vi "SEH Error Notification.vi"(6 "Configuration":T2, 7 "Command":T3, 8 "Error to Send":errorcluster, 11 "Priority":i32) -> (0 "Transmission Error":errorcluster, 1 "Transmitted Error":errorcluster, 2 "Empty?":bool, 3 "Priority Out":i32, 4 "Occurrences":i32, 5 "First Occurrence":timestamp)   [LabVIEW 2014]
uses:
  Controls/Shared/SEH Error Notification Command.ctl
  Controls/Shared/SEH Error Notification Config.ctl
  Controls/SEH/SEH Error Notification Data.ctl
  Controls/Shared/SEH Transmit Error Function.ctl
panel:
  out "Read Ptrs":i32[](array[numeric])
  out "Array":T1[][](array[typedef])
  out "Codes":i32[][](array[numeric])
  out "Sizes":i32[](array[numeric])
  out "Write Ptrs":i32[](array[numeric])
  # "Debug"
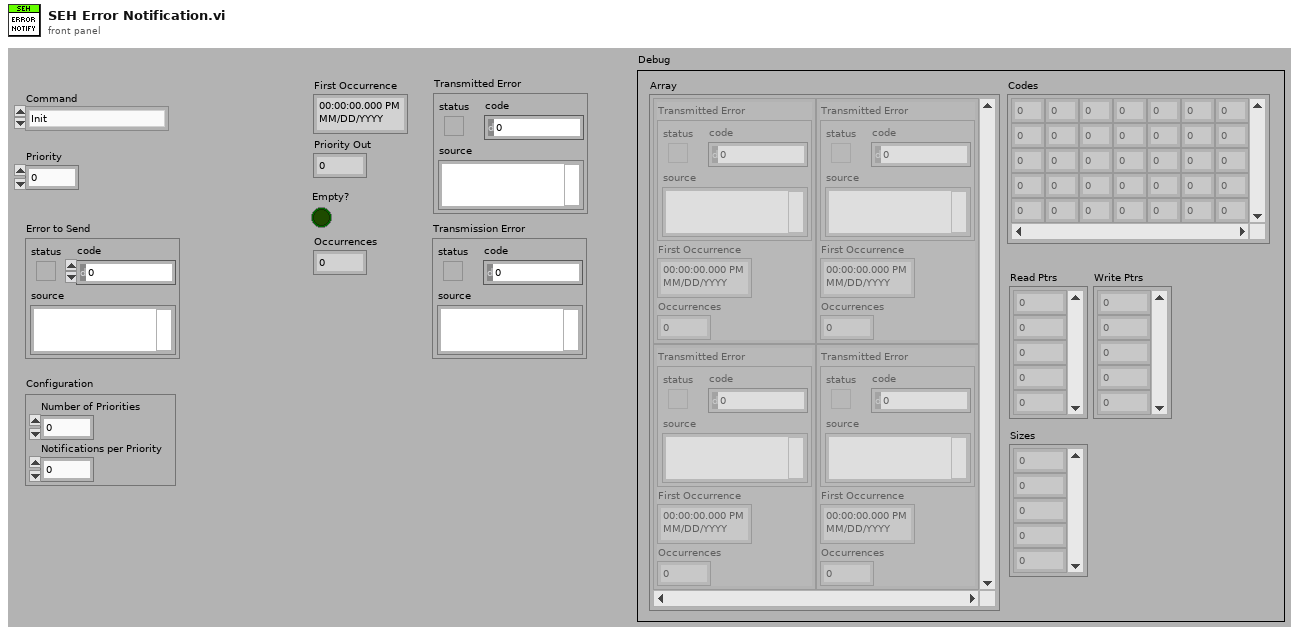
[diagram p1: front panel]
types:
  T1 = typedef "SEH Error Notification Data.ctl" = cluster{"Transmitted Error":errorcluster, "First Occurrence":timestamp, "Occurrences":i32}
  T2 = typedef "SEH Error Notification Config.ctl" = cluster{"Number of Priorities":i32, "Notifications per Priority":i32}
  T3 = typedef "SEH Error Notification Command.ctl" = enum16{"Init", "Send Error", "Check Error", "Invalid Command"}
  T4 = typedef "SEH Transmit Error Function.ctl" = enum8{"Set", "Reset", "No Change"}
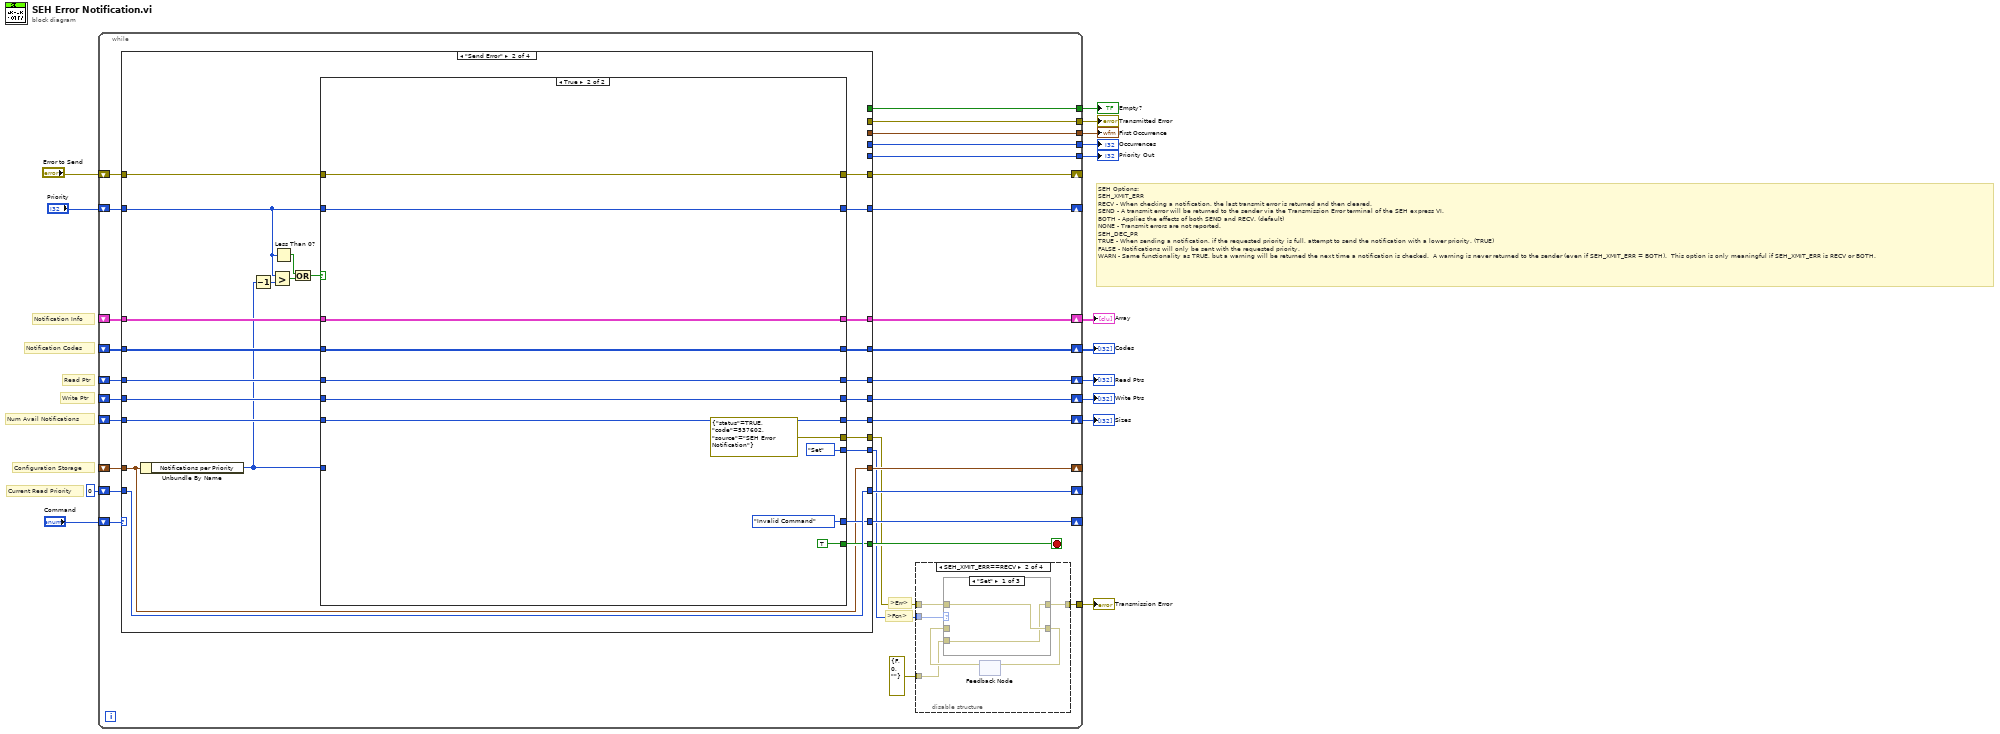
[diagram p0: block diagram]
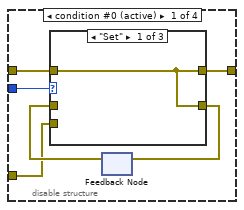
[diagram p2: hidden frame]
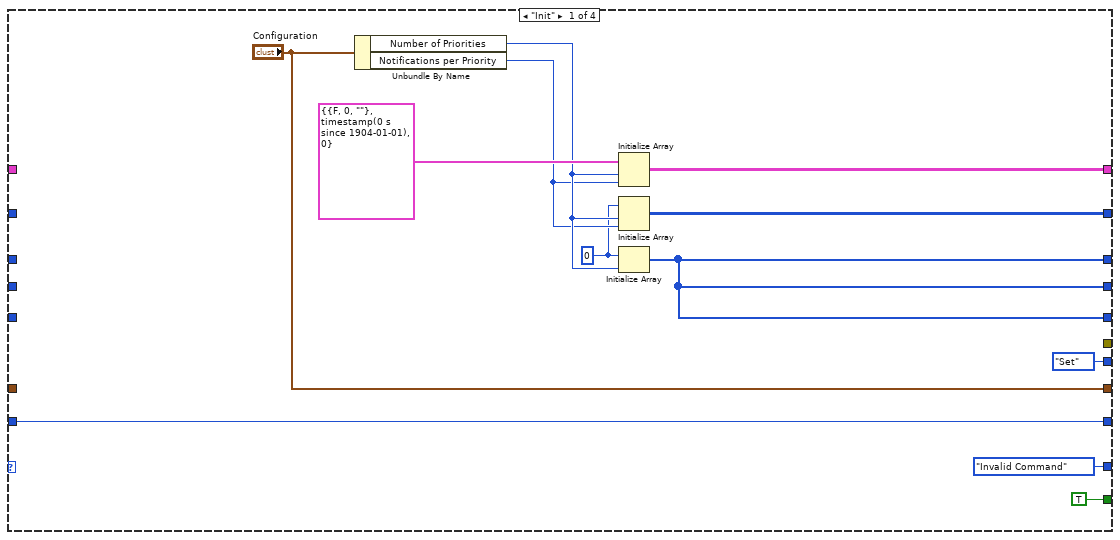
[diagram p9: hidden frame]
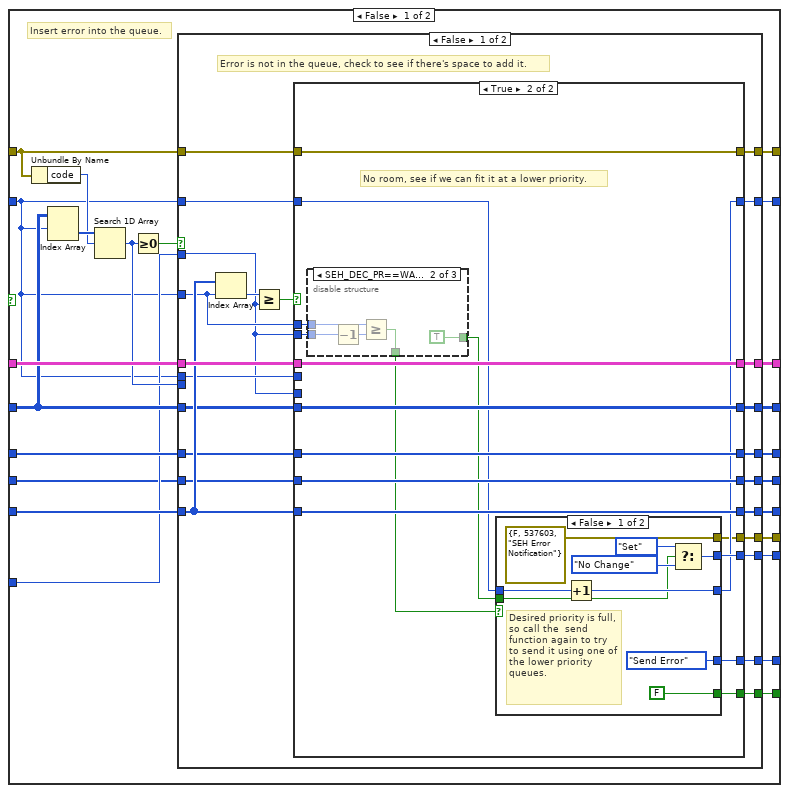
[diagram p10: hidden frame]
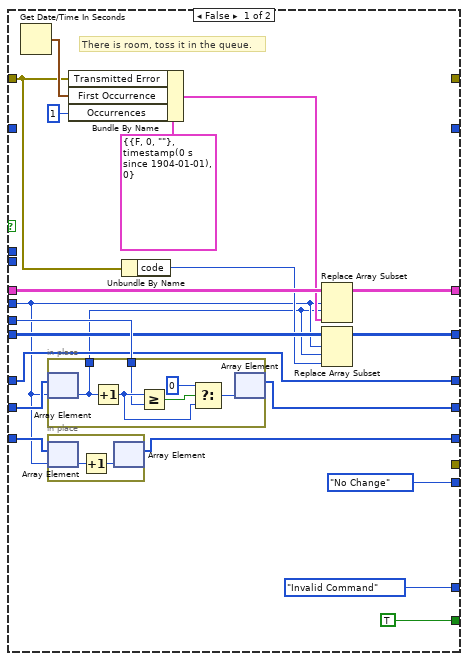
[diagram p11: hidden frame]
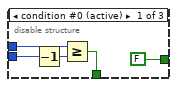
[diagram p12: hidden frame]
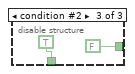
[diagram p13: hidden frame]
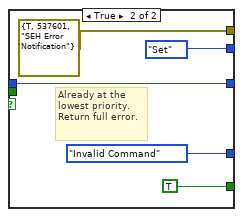
[diagram p14: hidden frame]
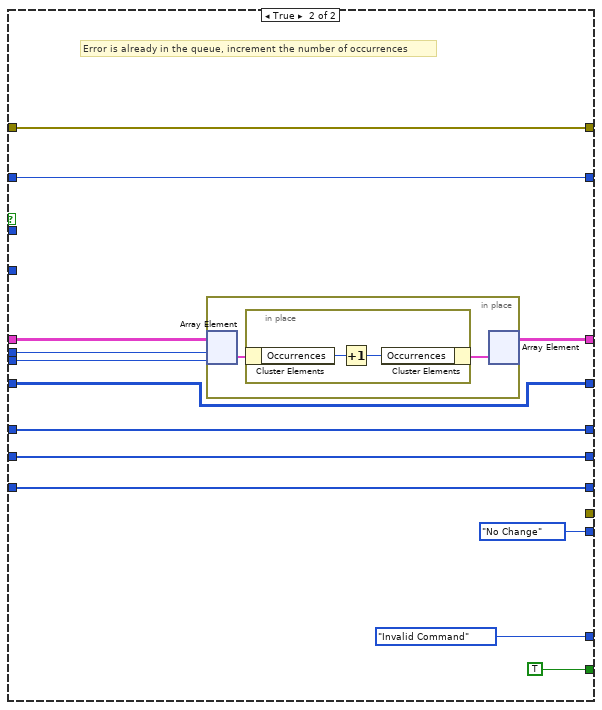
[diagram p15: hidden frame]
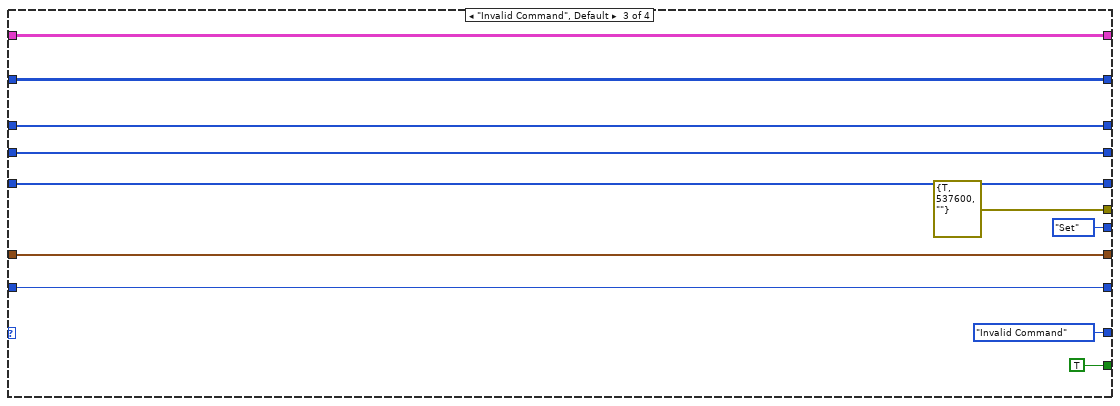
[diagram p16: hidden frame]
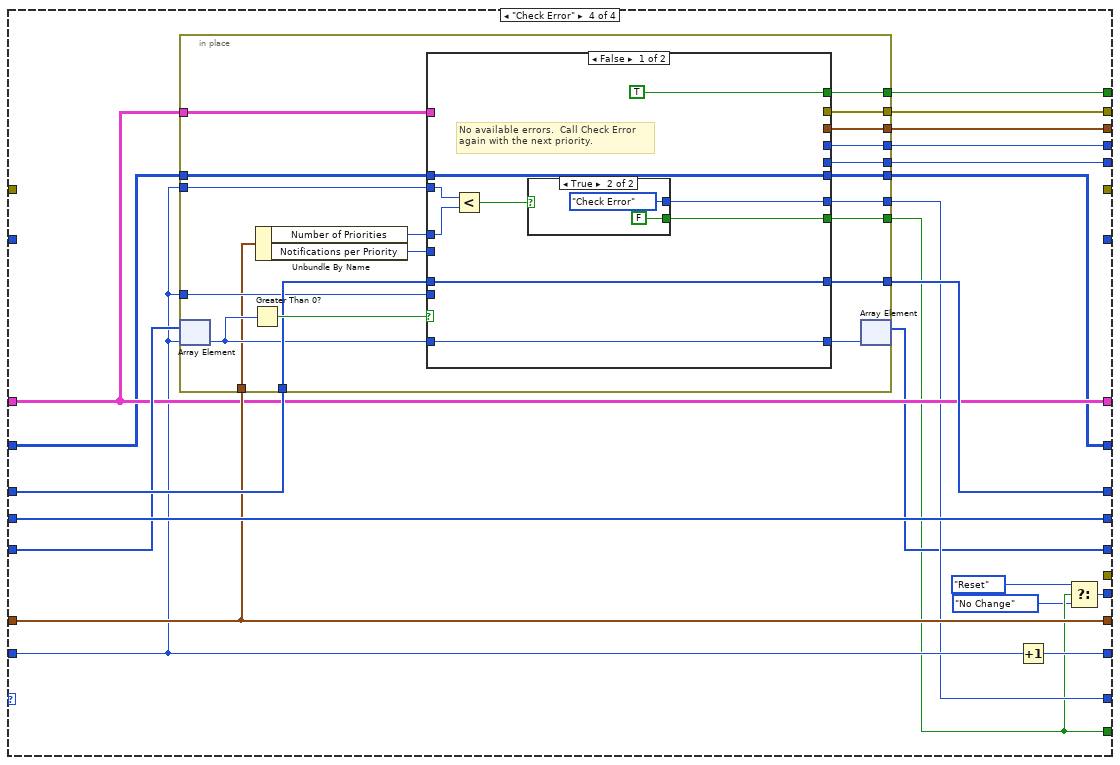
[diagram p17: hidden frame]
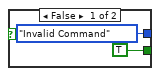
[diagram p18: hidden frame]
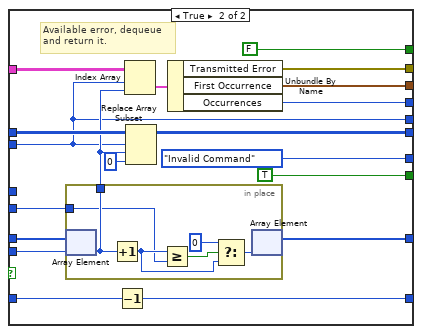
[diagram p19: hidden frame]
diagram:
  # "SEH Options:\nSEH_XMIT_ERR\nRECV - When checking a notification, the last transmit error is returned and then cleared.\nSEND - A transmit error will be returned to the sender via the Transmission Error terminal of the SEH express VI.\nBOTH - Applies the effects of both SEND and RECV. (default)\nNONE - Transmit errors are not reported.\nSEH_DEC_PR\nTRUE - When sending a notification, if the requested priority is full, attempt to send the notification with a lower priority. (TRUE)\nFALSE - Notifications will only be sent with the requested priority.\nWARN - Same functionality as TRUE, but a warning will be returned the next time a notification is checked.  A warning is never returned to the sender (even if SEH_XMIT_ERR = BOTH).  This option is only meaningful if SEH_XMIT_ERR is RECV or BOTH."
  # "Current Read Priority"
  # "Write Ptr"
  # "Configuration Storage"
  # "Notification Codes"
  # "Num Avail Notifications"
  # "Read Ptr"
  # "Notification Info"
  n1 = while {
    shift-right: [w44] -> w4
    shift-left: _ -> [w43]
    shift-right: [w42] -> w3
    shift-left: _ -> [w41]
    shift-right: [w40] -> w6
    shift-left: _ -> [w39]
    shift-right: [w38] -> _
    shift-left: _ -> [w37]
    shift-right: [w36] -> w5
    shift-left: _ -> [w35]
    shift-right: [w33] -> w7
    shift-left: _ -> [w32]
    shift-right: [w30] -> _
    shift-left: 0 -> [w31]
    shift-right: [w28] -> _
    shift-left: "Command" -> [w45]
    tunnel: [w27] -> w10
    tunnel: [w26] -> w11
    tunnel: [w25] -> w9
    tunnel: [w24] -> w8
    tunnel: [w23] -> w12
    shift-right: [w21] -> _
    shift-left: "Error to Send" -> [w34]
    shift-right: [w20] -> _
    shift-left: "Priority" -> [w22]
    tunnel: [w17] -> w1
    stop <- w29 stop-if-true
    # ">Err>"
    # ">Fcn>"
    n2 = case shown="\"Send Error\"" w45 {
      tunnel: [w81 w104 w263 w278] -> w44
      tunnel: w43 -> [_ w107 w263 w278]
      tunnel: [w75 w102 w262 w280] -> w42
      tunnel: w41 -> [_ w103 w262 w282]
      tunnel: [w75 w100 w261 w268] -> w40
      tunnel: w39 -> [_ w101 w261 w279]
      tunnel: ["Configuration" w91 w260 w281] -> w38
      tunnel: w37 -> [_ w91 w260 w281]
      tunnel: [w77 w105 w259 w272] -> w36
      tunnel: w35 -> [_ w106 w259 w277]
      tunnel: w34 -> [_ w99 _ _]
      tunnel: [w75 w97 w258 w284] -> w33
      tunnel: w32 -> [_ w98 w258 w284]
      tunnel: w31 -> [w74 w96 w257 w276]
      tunnel: [w74 w96 w257 w283] -> w30
      tunnel: [TRUE w95 TRUE w267] -> w29
      tunnel: [SEH_Error_Notification_Command."Invalid Command" ("Command") w94 SEH_Error_Notification_Command."Invalid Command" ("Command") w269] -> w28
      tunnel: [_ _ _ w275] -> w27
      tunnel: [_ _ _ w274] -> w26
      tunnel: [_ _ _ w273] -> w25
      tunnel: [_ _ _ w271] -> w24
      tunnel: [_ _ _ w270] -> w23
      tunnel: w22 -> [_ w88 _ _]
      tunnel: [_ w93 _ _] -> w21
      tunnel: [_ w92 _ _] -> w20
      tunnel: [_ w84 errorcluster {"status"=TRUE, "code"=537600, "source"=""} ("error out") _] -> w18
      tunnel: [SEH_Transmit_Error_Function."Set" w83 SEH_Transmit_Error_Function."Set" w264] -> w19
      frame "Init" {
        w78 = 0
        n3 = Unbundle By Name("Configuration") -> ("Number of Priorities"=w80:i32, "Notifications per Priority"=w79:i32)
        n4 = Initialize Array(T1 {"Transmitted Error"={"status"=FALSE, "code"=0, "source"=""}, "First Occurrence"=timestamp(0 s since 1904-01-01), "Occurrences"=0} ("Error Info"), w80, w79) -> (w81:T1[][])
        n5 = Initialize Array(w78, w80, w79) -> (w77:i32[][])
        n6 = Initialize Array(w78, w80) -> (w75:i32[])
      }
      frame "Send Error" {
        n7 = Unbundle By Name(w91) -> ("Notifications per Priority"=w90:i32)
        n8 = Decrement(x=w90) -> (x-1=w89:i32)
        n9 = Greater?(x=w88, y=w89) -> (0:w87:bool)
        n10 = Less Than 0?(x=w88) -> (x < 0?=w86:bool)
        n11 = Or(x=w86, y=w87) -> (x .or. y?=w85:bool)
        n12 = case shown="True" w85 {
          tunnel: w107 -> [w127 w245]
          tunnel: w106 -> [w125 w246]
          tunnel: [w124 w246] -> w105
          tunnel: [w123 w245] -> w104
          tunnel: w103 -> [w122 w247]
          tunnel: [w121 w247] -> w102
          tunnel: w101 -> [w120 w249]
          tunnel: [w119 w249] -> w100
          tunnel: w90 -> [w118 _]
          tunnel: w99 -> [w117 w252]
          tunnel: w98 -> [w116 w248]
          tunnel: [w115 w248] -> w97
          tunnel: [w114 TRUE] -> w95
          tunnel: [w113 SEH_Error_Notification_Command."Invalid Command" ("Command")] -> w94
          tunnel: [w112 w252] -> w93
          tunnel: w88 -> [w111 w244]
          tunnel: [w110 w244] -> w92
          tunnel: [w109 SEH_Transmit_Error_Function."Set"] -> w83
          tunnel: [w108 errorcluster {"status"=TRUE, "code"=537602, "source"="SEH Error Notification"} ("error out")] -> w84
          frame False {
            # "Insert error into the queue."
            n13 = Unbundle By Name(w117) -> ("code"=w129:i32)
            n14 = Index Array(array=w125, index (row)=w111) -> (element=w130:i32[])  [unwired: 1 in]
            n15 = Search 1D Array(1D array=w130, element=w129) -> (index of element=w126:i32)  [unwired: 1 in]
            n16 = Greater Or Equal To 0?(x=w126) -> (x >= 0?=w128:bool)
            n17 = case shown="False" w128 {
              tunnel: w127 -> [w151 w237]
              tunnel: w111 -> [w141 w236]
              tunnel: w126 -> [_ w235]
              tunnel: w125 -> [w144 w234]
              tunnel: [w143 w234] -> w124
              tunnel: [w150 w233] -> w123
              tunnel: w122 -> [w146 w232]
              tunnel: [w145 w232] -> w121
              tunnel: w120 -> [w148 w231]
              tunnel: [w147 w231] -> w119
              tunnel: [w149 SEH_Transmit_Error_Function."No Change"] -> w109
              tunnel: w118 -> [w132 _]
              tunnel: w117 -> [w142 w228]
              tunnel: w116 -> [w140 w230]
              tunnel: [w139 w230] -> w115
              tunnel: w111 -> [w136 _]
              tunnel: [w138 TRUE] -> w114
              tunnel: [w137 SEH_Error_Notification_Command."Invalid Command" ("Command")] -> w113
              tunnel: [w135 w228] -> w112
              tunnel: w111 -> [w134 w227]
              tunnel: [w133 w227] -> w110
              tunnel: [w131 _] -> w108
              frame False {
                # "Error is not in the queue, check to see if there's space to add it."
                n18 = Index Array(array=w148, index=w136) -> (element=w153:i32)
                n19 = Greater Or Equal?(x=w153, y=w132) -> (x >= y?=w152:bool)
                n20 = case shown="True" w152 {
                  tunnel: w151 -> [w174 w198]
                  tunnel: [w173 w198] -> w150
                  tunnel: [SEH_Transmit_Error_Function."No Change" w197] -> w149
                  tunnel: w148 -> [w168 w196]
                  tunnel: [w167 w196] -> w147
                  tunnel: [w163 w195] -> w145
                  tunnel: w146 -> [w163 w195]
                  tunnel: w144 -> [w162 w194]
                  tunnel: [w161 w194] -> w143
                  tunnel: w142 -> [w160 w188]
                  tunnel: w141 -> [w158 _]
                  tunnel: w140 -> [w165 w193]
                  tunnel: [w166 w193] -> w139
                  tunnel: w132 -> [w164 _]
                  tunnel: [TRUE w192] -> w138
                  tunnel: [SEH_Error_Notification_Command."Invalid Command" ("Command") w191] -> w137
                  tunnel: w136 -> [_ w190]
                  tunnel: w132 -> [_ w185]
                  tunnel: [_ w188] -> w135
                  tunnel: w134 -> [_ w187]
                  tunnel: [_ w186] -> w133
                  tunnel: [_ w184] -> w131
                  frame False {
                    # "There is room, toss it in the queue."
                    n21 = Get Date/Time In Seconds() -> (seconds since 1Jan1904=w169:timestamp)
                    n22 = in-place {
                      in-place-border: [w176] -> w157
                      in-place-border: w164 -> [w175]
                      n23 = in-place-array #1(w165, w158) -> (w176:i32)
                      n24 = Increment(x=w176) -> (x+1=w179:i32)
                      n25 = Greater Or Equal?(x=w179, y=w175) -> (x >= y?=w180:bool)
                      n26 = Select(t=0, s=w180, f=w179) -> (s? t:f=w177:i32)
                      n27 = in-place-array #1(w177) -> (w166:i32[])  [unwired: 1 out]
                    }
                    n28 = in-place {
                      n29 = in-place-array #2(w168, w158) -> (w182:i32)
                      n30 = Increment(x=w182) -> (x+1=w181:i32)
                      n31 = in-place-array #2(w181) -> (w167:i32[])  [unwired: 1 out]
                    }
                    n32 = Bundle By Name(cluster=T1 {"Transmitted Error"={"status"=FALSE, "code"=0, "source"=""}, "First Occurrence"=timestamp(0 s since 1904-01-01), "Occurrences"=0} ("Error Info"), "Transmitted Error"=w160, "First Occurrence"=w169, "Occurrences"=1) -> (w170:T1)
                    n33 = Unbundle By Name(w160) -> ("code"=w159:i32)
                    n34 = Replace Array Subset(array=w174, new element=w170, index (row)=w158, index (col)=w157) -> (w173:T1[][])
                    n35 = Replace Array Subset(array=w162, new element=w159, index (row)=w158, index (col)=w157) -> (w161:i32[][])
                  }
                  frame True {
                    # "No room, see if we can fit it at a lower priority."
                    n36 = disable-structure shown="SEH_DEC_PR==WARN" {
                      disable-tunnel: w190 -> [w203 w208 _]
                      disable-tunnel: [w202 w207 TRUE] -> w189
                      disable-tunnel: w185 -> [w201 w206 _]
                      disable-tunnel: [FALSE TRUE FALSE] -> w183
                      frame condition #0 (active) {
                        n37 = Decrement(x=w201) -> (x-1=w200:i32)
                        n38 = Greater Or Equal?(x=w203, y=w200) -> (x >= y?=w202:bool)
                      }
                      frame condition #1 {
                        n39 = Decrement(x=w206) -> (x-1=w205:i32)
                        n40 = Greater Or Equal?(x=w208, y=w205) -> (x >= y?=w207:bool)
                      }
                      frame condition #2 {
                      }
                    }
                    n41 = case shown="False" w189 {
                      tunnel: [w213 SEH_Transmit_Error_Function."Set"] -> w197
                      tunnel: [FALSE TRUE] -> w192
                      tunnel: [SEH_Error_Notification_Command."Send Error" ("Command") SEH_Error_Notification_Command."Invalid Command" ("Command")] -> w191
                      tunnel: w187 -> [w219 w222]
                      tunnel: [w218 w222] -> w186
                      tunnel: [errorcluster {"status"=FALSE, "code"=537603, "source"="SEH Error Notification"} ("error out") errorcluster {"status"=TRUE, "code"=537601, "source"="SEH Error Notification"} ("error out")] -> w184
                      tunnel: w183 -> [w212 _]
                      frame False {
                        # "Desired priority is full, so call the  send function again to try to send it using one of the lower priority queues."
                        n42 = Increment(x=w219) -> (x+1=w218:i32)
                        n43 = Select(t=SEH_Transmit_Error_Function."Set", s=w212, f=SEH_Transmit_Error_Function."No Change") -> (s? t:f=w213:T4)
                      }
                      frame True {
                        # "Already at the lowest priority.\nReturn full error."
                      }
                    }
                  }
                }
              }
              frame True {
                # "Error is already in the queue, increment the number of occurrences"
                # "Error is already in the queue, increase # of occurrences"
                n44 = in-place {
                  n45 = in-place-array #3(w237, w236, w235) -> (w239:T1)
                  n46 = in-place {
                    n47 = in-place-cluster #4(w239) -> ("Occurrences"=w241:i32)
                    n48 = Increment(x=w241) -> (x+1=w240:i32)
                    n49 = in-place-cluster #4("Occurrences"=w240) -> (w238:T1)
                  }
                  n50 = in-place-array #3(w238) -> (w233:T1[][])  [unwired: 2 out]
                }
              }
            }
          }
          frame True {
          }
        }
      }
      frame "Invalid Command", Default {
      }
      frame "Check Error" {
        n51 = in-place {
          in-place-border: w282 -> [w303]
          in-place-border: w281 -> [w287]
          in-place-border: [w302] -> w280
          in-place-border: w276 -> [w301]
          in-place-border: w278 -> [w297]
          in-place-border: w277 -> [w298]
          in-place-border: w276 -> [w296]
          in-place-border: [w295] -> w275
          in-place-border: [w294] -> w274
          in-place-border: [w293] -> w273
          in-place-border: [w292] -> w272
          in-place-border: [w291] -> w271
          in-place-border: [w290] -> w270
          in-place-border: [w289] -> w269
          in-place-border: [w288] -> w267
          n52 = in-place-array #5(w279, w276) -> (w300:i32)
          n53 = Greater Than 0?(x=w300) -> (x > 0?=w304:bool)
          n54 = Unbundle By Name(w287) -> ("Number of Priorities"=w285:i32, "Notifications per Priority"=w286:i32)
          n55 = case shown="False" w304 {
            tunnel: w303 -> [w312 w336]
            tunnel: [w312 w335] -> w302
            tunnel: w301 -> [_ w334]
            tunnel: w300 -> [w313 w333]
            tunnel: [w313 w332] -> w299
            tunnel: w298 -> [w311 w331]
            tunnel: w297 -> [_ w329]
            tunnel: w296 -> [w307 w322]
            tunnel: [_ w326] -> w295
            tunnel: [_ w325] -> w294
            tunnel: [_ w324] -> w293
            tunnel: [w311 w323] -> w292
            tunnel: [_ w322] -> w291
            tunnel: [TRUE FALSE] -> w290
            tunnel: [w309 SEH_Error_Notification_Command."Invalid Command" ("Command")] -> w289
            tunnel: [w308 TRUE] -> w288
            tunnel: w286 -> [_ w318]
            tunnel: w285 -> [w306 _]
            frame False {
              # "No available errors.  Call Check Error \nagain with the next priority."
              n56 = Less?(x=w307, y=w306) -> (x < y?=w305:bool)
              n57 = case shown="True" w305 {
                tunnel: [SEH_Error_Notification_Command."Invalid Command" ("Command") SEH_Error_Notification_Command."Check Error" ("Command")] -> w309
                tunnel: [TRUE FALSE] -> w308
                frame False {
                }
                frame True {
                }
              }
            }
            frame True {
              # "Available error, dequeue \nand return it."
              n58 = in-place {
                in-place-border: [w338] -> w328
                in-place-border: w318 -> [w337]
                n59 = in-place-array #6(w336, w334) -> (w338:i32)
                n60 = Increment(x=w338) -> (x+1=w341:i32)
                n61 = Greater Or Equal?(x=w341, y=w337) -> (x >= y?=w342:bool)
                n62 = Select(t=0, s=w342, f=w341) -> (s? t:f=w339:i32)
                n63 = in-place-array #6(w339) -> (w335:i32[])  [unwired: 1 out]
              }
              n64 = Decrement(x=w333) -> (x-1=w332:i32)
              n65 = Index Array(array=w329, index (row)=w322, index (col)=w328) -> (element=w327:T1)
              n66 = Replace Array Subset(array=w331, new element=0 ("new element/subarray"), index (row)=w322, index (col)=w328) -> (w323:i32[][])
              n67 = Unbundle By Name(w327) -> ("Transmitted Error"=w326:errorcluster, "First Occurrence"=w325:timestamp, "Occurrences"=w324:i32)
            }
          }
          n68 = in-place-array #5(w299) -> (w268:i32[])  [unwired: 1 out]
        }
        n69 = Increment(x=w276) -> (x+1=w283:i32)
        n70 = Select(t=SEH_Transmit_Error_Function."Reset", s=w267, f=SEH_Transmit_Error_Function."No Change") -> (s? t:f=w264:T4)
      }
    }
    n71 = disable-structure shown="SEH_XMIT_ERR==RECV" {
      disable-tunnel: w18 -> [w50 w61 w69 _]
      disable-tunnel: w19 -> [w51 w62 _ _]
      disable-tunnel: [w47 w58 w69 w70] -> w17
      disable-tunnel: errorcluster {"status"=FALSE, "code"=0, "source"=""} ("error out") -> [w46 w57 _ w70]
      frame condition #0 (active) {
        n72 = feedback #7() -> (w48:errorcluster)  [unwired: 1 in]
        n73 = case shown="\"Set\"" w51 {
          tunnel: w50 -> [w52 _ _]
          tunnel: w46 -> [_ w54 w55]
          tunnel: [w52 w54 w56] -> w49
          tunnel: w48 -> [_ w53 w56]
          tunnel: [w52 w53 w55] -> w47
          frame "Set" {
          }
          frame "Reset" {
          }
          frame "No Change", Default {
          }
        }
        n74 = feedback-in #7(w49) -> ()
      }
      frame condition #1 {
        n75 = feedback #8() -> (w59:errorcluster)  [unwired: 1 in]
        n76 = case shown="\"Set\"" w62 {
          tunnel: w61 -> [w64 _ _]
          tunnel: w57 -> [w63 w66 w67]
          tunnel: [w64 w66 w68] -> w60
          tunnel: w59 -> [_ w65 w68]
          tunnel: [w63 w65 w67] -> w58
          frame "Set" {
          }
          frame "Reset" {
          }
          frame "No Change", Default {
          }
        }
        n77 = feedback-in #8(w60) -> ()
      }
      frame condition #2 {
      }
      frame condition #3 {
      }
    }
  }
  "Empty?" <- w12
  "Priority Out" <- w8
  "First Occurrence" <- w11
  "Occurrences" <- w9
  "Transmitted Error" <- w10
  "Write Ptrs" <- w7
  "Sizes" <- w6
  "Codes" <- w5
  "Array" <- w4
  "Read Ptrs" <- w3
  "Transmission Error" <- w1
